vi "Arcade Drive.vi"(10 "Turn Power":dbl, 11 "Y Power":dbl) -> (2 "Right Motor Output":dbl, 3 "Left Motor Output":dbl)   [LabVIEW 2017]
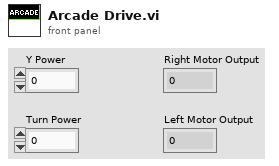
[diagram p1: front panel]
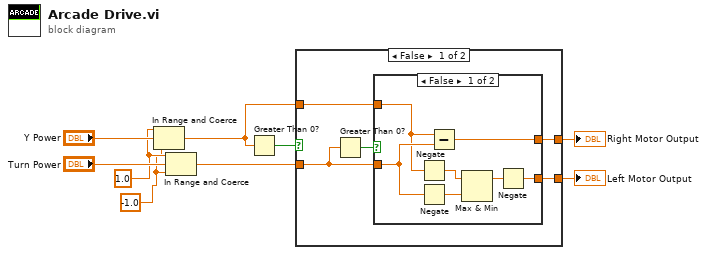
[diagram p0: block diagram]
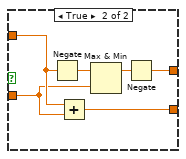
[diagram p2: hidden frame]
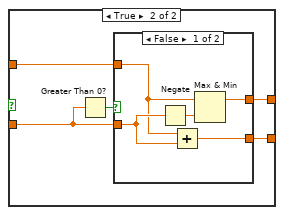
[diagram p3: hidden frame]
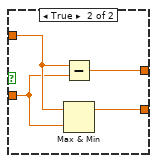
[diagram p4: hidden frame]
diagram:
  w2 = 1.0 ("upper limit")
  w1 = -1.0 ("lower limit")
  n1 = In Range and Coerce(upper limit=w2, x="Y Power", lower limit=w1) -> (coerced(x)=w4:dbl)  [unwired: 1 out]
  n2 = In Range and Coerce(upper limit=w2, x="Turn Power", lower limit=w1) -> (coerced(x)=w3:dbl)  [unwired: 1 out]
  n3 = Greater Than 0?(x=w4) -> (x > 0?=w9:bool)
  n4 = case shown="False" w9 {
    tunnel: w3 -> [w13 w31]
    tunnel: w4 -> [w12 w30]
    tunnel: [w11 w29] -> w6
    tunnel: [w10 w28] -> w5
    frame False {
      n5 = Greater Than 0?(x=w13) -> (x > 0?=w14:bool)
      n6 = case shown="False" w14 {
        tunnel: w13 -> [w21 w23]
        tunnel: w12 -> [w19 w24]
        tunnel: [w15 w25] -> w11
        tunnel: [w16 w22] -> w10
        frame False {
          n7 = Negate(x=w19) -> (-x=w20:dbl)
          n8 = Negate(x=w21) -> (-x=w18:dbl)
          n9 = Subtract(x=w19, y=w21) -> (x-y=w15:dbl)
          n10 = Max & Min(x=w20, y=w18) -> (max(x,y)=w17:dbl)  [unwired: 1 out]
          n11 = Negate(x=w17) -> (-x=w16:dbl)
        }
        frame True {
          n12 = Negate(x=w24) -> (-x=w27:dbl)
          n13 = Add(x=w24, y=w23) -> (x+y=w22:dbl)
          n14 = Max & Min(x=w27, y=w23) -> (max(x,y)=w26:dbl)  [unwired: 1 out]
          n15 = Negate(x=w26) -> (-x=w25:dbl)
        }
      }
    }
    frame True {
      n16 = Greater Than 0?(x=w31) -> (x > 0?=w32:bool)
      n17 = case shown="False" w32 {
        tunnel: w31 -> [w37 w39]
        tunnel: w30 -> [w34 w40]
        tunnel: [w35 w38] -> w29
        tunnel: [w33 w41] -> w28
        frame False {
          n18 = Negate(x=w37) -> (-x=w36:dbl)
          n19 = Add(x=w34, y=w37) -> (x+y=w33:dbl)
          n20 = Max & Min(x=w34, y=w36) -> (max(x,y)=w35:dbl)  [unwired: 1 out]
        }
        frame True {
          n21 = Subtract(x=w40, y=w39) -> (x-y=w38:dbl)
          n22 = Max & Min(x=w40, y=w39) -> (max(x,y)=w41:dbl)  [unwired: 1 out]
        }
      }
    }
  }
  "Right Motor Output" <- w6
  "Left Motor Output" <- w5
